vi "iRobot Navigation Target.vi"() -> ()   [LabVIEW 2015]
uses:
  iRobot/Sensor/OI Mode.ctl
  iRobot/Sensor/Charging Sources Available.ctl
  iRobot/Sensor/Cargo Bay Digital Inputs.ctl
  iRobot/Sensor/Charging State.ctl
  iRobot/Sensor/Buttons.ctl
  iRobot/Sensor/Low-Side Driver + Wheel Overcurrent.ctl
  iRobot/Sensor/Bumps + Wheel Drops.ctl
  <vilib>/Statechart/Infrastructure/RTStatechart/RunTime SCN.xnode
  iRobot/Sensor/Sensor Group 6.ctl
  Accelerometer.ctl
  iRobot Navigation State Machine.lvsc
  iRobot Navigation State Machine.lvsc/Inputs.ctl
  iRobot Navigation State Machine.lvsc/Outputs.ctl
  iRobot Navigation State Machine.lvsc/Trigger.ctl
  iRobot Navigation State Machine.lvsc/State.ctl
  iRobot Navigation State Machine.lvsc/StatechartState.ctl
  <vilib>/myRIO/Instrument Drivers/Utilities/Utilities.lvlib
  iRobot Navigation State Machine.lvsc/CompanionDiagram.vi
  iRobot Navigation State Machine.lvsc/CompanionDiagram.vi/52/SC Main.vi
  <vilib>/myRIO/Express VI/Onboard IO/I2C/I2C Express VI.xnode
  <vilib>/myRIO/Instrument Drivers/Onboard IO/I2C/vis/Configure.vi
  <vilib>/myRIO/Instrument Drivers/Onboard IO/I2C/I2C.lvlib
  <vilib>/myRIO/Instrument Drivers/Onboard IO/I2C/typedefs/I2C Transfer Rate.ctl
  <vilib>/myRIO/Instrument Drivers/Onboard IO/I2C/typedefs/I2C User Configuration.ctl
  <vilib>/myRIO/Instrument Drivers/Onboard IO/I2C/typedefs/I2C Configuration.ctl
  <vilib>/myRIO/Common/Instrument Driver Framework/myRIO v1.0/I2C/typedefs/I2C Channels Enum.ctl
  <vilib>/myRIO/Common/Instrument Driver Framework/Utilities/typedefs/Generic FPGA Reference.ctl
  <vilib>/myRIO/Common/Instrument Driver Framework/Utilities/typedefs/myRIO v1.0 Reference.ctl
  <vilib>/myRIO/Common/Instrument Driver Framework/Utilities/typedefs/Hardware Version Enum.ctl
  <vilib>/myRIO/Common/Instrument Driver Framework/Utilities/typedefs/myRIO Generic Hardware Reference.ctl
  <vilib>/myRIO/Instrument Drivers/Onboard IO/I2C/typedefs/I2C Reference.ctl
  <vilib>/myRIO/Instrument Drivers/Onboard IO/I2C/vis/myRIO I2C Open.xnode
  <vilib>/myRIO/Common/Instrument Driver Framework/Utilities/vis/Is FPGA Ref Available.vi
  <vilib>/myRIO/Common/Instrument Driver Framework/myRIO v1.0/I2C/vis/myRIO v1.1 Open I2C.vi
  <vilib>/userdefined/High Color/nirio_resource_hc.ctl
  iRobot Sensors.ctl
panel:
  out "StateData.Speed":i16
  in  "Tab Control":T1(tab)
  out "Right Wheel":i16
  out "Left Wheel":i16
  out "PID output":dbl
  in  "Kd Constant":dbl
  in  "Ki Constant":dbl=30.0
  in  "Kp Constant":dbl=350.0
  out "Current barcode time":dbl
  in  "Barcode Response\nTime Delay":dbl=0.5
  in  "Barcode Time Threshold \n(to measure lenght of each line":dbl=0.45
  in  "Barcode Tape \nSensor Threshold":u16=600
  out "iRobot Sensors (graphical)":T2 {"Right Wheel (mm/s)" scale=-500.0..500.0; "Left Wheel (mm/s)" scale=-500.0..500.0}
  in  "Edge Tape\nSensor Threshold":u16=600
  out "Barcode Array":i32[](array[numeric])
  out "Active States":T4
  out "error out":errorcluster
  in  "Wheel Speed (mm/s)":i16(slide)=100 scale=0.0..500.0
  in  "accel smoothing (0-1)":dbl=0.1
  in  "stop":bool
  out "Target Running":bool
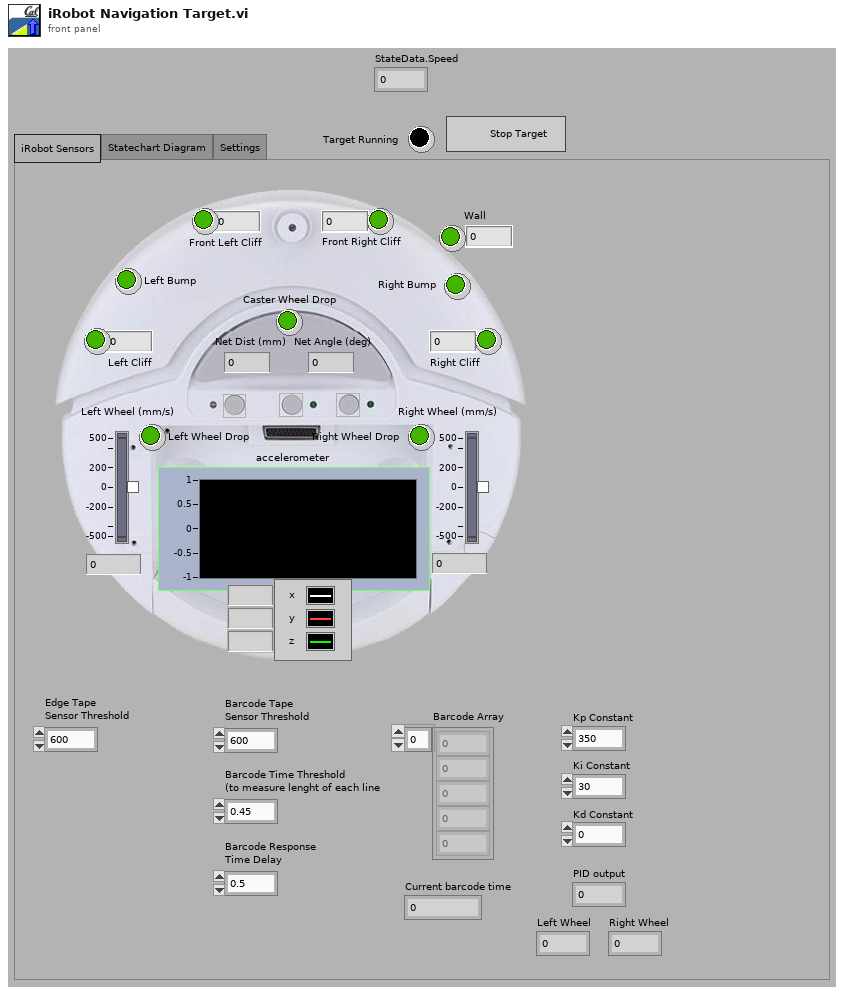
[diagram p1: front panel]
types:
  T1 = enum32{"iRobot Sensors", "Statechart Diagram", "Settings"}
  T2 = typedef "iRobot Sensors.ctl" = cluster{"Caster Wheel Drop":bool, "Left Wheel Drop":bool, "Right Wheel Drop":bool, "Left Bump":bool, "Right Bump":bool, "Left Cliff":bool, "Front Left Cliff":bool, "Front Right Cliff":bool, "Right Cliff":bool, "Wall":bool, "Net Dist (mm)":i32, "Net Angle (deg)":i32, "Wall":u16, "Left Cliff":u16, "Front Left Cliff":u16, "Front Right Cliff":u16, "Right Cliff":u16, "Left Wheel (mm/s)":i16, "Right Wheel (mm/s)":i16, "accelerometer":T3}
  T3 = typedef "Accelerometer.ctl" = cluster{"x axis (g)":dbl, "y axis (g)":dbl, "z axis (g)":dbl}
  T4 = typedef "iRobot Navigation State Machine.lvsc/StatechartState.ctl" = T5[]
  T5 = typedef "iRobot Navigation State Machine.lvsc/State.ctl" = enum16{"NI.SC.Initial", "NI.SC.History", "NI.SC.ShallowHistory", "NI.SC.Terminal", "Pause", "Run", "Pause\\Detect Play Button\\Pause;\nWait for\nbutton\nrelease", "Pause\\Detect Play Button\\Unpause;\nwait for\nbutton release", "Pause\\Detect Play Button\\Unpause;\nwait for\nbutton press", "Run\\Detect Obstacles\\Recover from head on\nedge collision", "Run\\Detect Obstacles\\Check barcode or edge", "Run\\Detect Obstacles\\Right Bumper", "Run\\Detect Obstacles\\Clear the barcode 2", "Run\\Detect Obstacles\\Clear the barcode", "Run\\Detect Obstacles\\Left Bumper", "Run\\Detect Obstacles\\Slow Down", "Run\\Detect Obstacles\\Speed Up", "Run\\Detect Obstacles\\Turn Right", "Run\\Detect Obstacles\\Turn Left", "Run\\Detect Obstacles\\Light", "Run\\Detect Obstacles\\Dark", "Run\\Detect Obstacles\\Straighten Left", "Run\\Detect Obstacles\\Straighten Right", "Run\\Detect Obstacles\\Barcode Drive", "Run\\Detect Obstacles\\Hit Right Boundary /\n Turn Left", "Run\\Detect Obstacles\\Hit Left Boundary / \nTurn Right", "Run\\Detect Obstacles\\Drive"}
  T6 = typedef "iRobot UART Port Type.ctl" = refnum<visa-resource-name>
  T7 = typedef "I2C.lvlib/I2C Reference.ctl" = cluster{"myRIO Reference":T8, "I2C Channels Enum":T12, "I2C Configuration":T13}
  T8 = typedef "myRIO Generic Hardware Reference.ctl" = cluster{"myRIO Model":T9, "myRIO Hardware Reference":T10}
  T9 = typedef "Hardware Version Enum.ctl" = enum16{"Unknown", "myRIO-1900", "myRIO-1950", "roboRIO"}
  T10 = typedef "myRIO v1.0 Reference.ctl" = cluster{"Generic FPGA Reference":T11, "Allow multiple opens":bool}
  T11 = typedef "Generic FPGA Reference.ctl" = refnum<k20>
  T12 = typedef "I2C Channels Enum.ctl" = enum16{"Not Connected", "A/I2C", "B/I2C", "I2C/I2C"}
  T13 = typedef "I2C.lvlib/I2C Configuration.ctl" = cluster{"I2C Transfer Rate":T14}
  T14 = typedef "I2C.lvlib/I2C Transfer Rate.ctl" = enum16{"Standard mode (100 kbps)", "Fast mode (400 kbps)"}
  T15 = typedef "I2C.lvlib/I2C User Configuration.ctl" = cluster{"I2C Transfer Rate":T14}
  T16 = typedef "nirio_resource_hc.ctl" = tag
  T17 = typedef "iRobot Navigation State Machine.lvsc/Inputs.ctl" = cluster{"net distance (mm)":i32, "net angle (deg)":i32, "Max Wheel Speed (mm/s)":i16, "accelerometer":T3, "iRobot Sensors":T18, "Is Simulator?":bool, "Edge Tape Threshold":u16, "Barcode Tape Threshold":u16, "Barcode Time Threshold":dbl, "Barcode Action Time":dbl, "Kp Constant":dbl, "Ki Constant":dbl, "Kd Constant":dbl}
  T18 = typedef "Sensor Group 6.ctl" = cluster{"Bumps + Wheel Drops":T19, "Wall":bool, "Cliff Left":bool, "Cliff Front Left":bool, "Cliff Front Right":bool, "Cliff Right":bool, "Virtual Wall":bool, "Low-Side Driver + Wheel Overcurrent":T20, "Infrared":u8, "Buttons":T21, "Distance (mm)":i32, "Angle (deg)":i32, "Charging State":T22, "Voltage (mV)":u16, "Current (mA)":i16, "Battery Temperature (deg C)":i8, "Battery Charge (mAh)":u16, "Battery Capacity (mAh)":u16, "Wall Signal (0-4095)":u16, "Cliff Left Signal (0-4095)":u16, "Cliff Front Left Signal (0-4095)":u16, "Cliff Front Right Signal (0-4095)":u16, "Cliff Right Signal (0-4095)":u16, "Cargo Bay Digital Inputs":T23, "Cargo Bay Analog Signal (0-1023)":u16, "Charging Sources Available":T24, "OI Mode":T25, "Song Number":u8, "Song Playing":bool, "Number of Stream Packets":u8, "Requested Velocity (mm/s)":i16, "Requested Radius (mm)":i16, "Requested Right Wheel Velocity (mm/s)":i16, "Requested Left Wheel Velocity (mm/s)":i16}
  T19 = typedef "Bumps + Wheel Drops.ctl" = cluster{"Wheeldrop Caster":bool, "Wheeldrop Left":bool, "Wheeldrop Right":bool, "Bump Left":bool, "Bump Right":bool}
  T20 = typedef "Low-Side Driver + Wheel Overcurrent.ctl" = cluster{"Low-Side Driver 0":bool, "Low-Side Driver 1":bool, "Low-Side Driver 2":bool, "Left Wheel":bool, "Right Wheel":bool}
  T21 = typedef "Buttons.ctl" = cluster{"Advance":bool, "Play":bool}
  T22 = typedef "Charging State.ctl" = enum16{"Not Charging", "Reconditioning Charging", "Full Charging", "Trickle Charging", "Waiting", "Charging Fault Condition"}
  T23 = typedef "Cargo Bay Digital Inputs.ctl" = cluster{"Digital Input 0":bool, "Digital Input 1":bool, "Digital Input 2":bool, "Digital Input 3":bool, "Device Detect":bool}
  T24 = typedef "Charging Sources Available.ctl" = cluster{"Internal Charger":bool, "Home Base":bool}
  T25 = typedef "OI Mode.ctl" = enum16{"Off", "Passive", "Safe", "Full"}
  T26 = typedef "iRobot Navigation State Machine.lvsc/Outputs.ctl" = cluster{"Left Wheel Speed (mm/s)":i16, "Right Wheel Speed (mm/s)":i16, "Current time":dbl, "Array":i32[], "PID output":dbl, "Left wheel":i16, "Right wheel":i16, "StateData.Speed":i16}
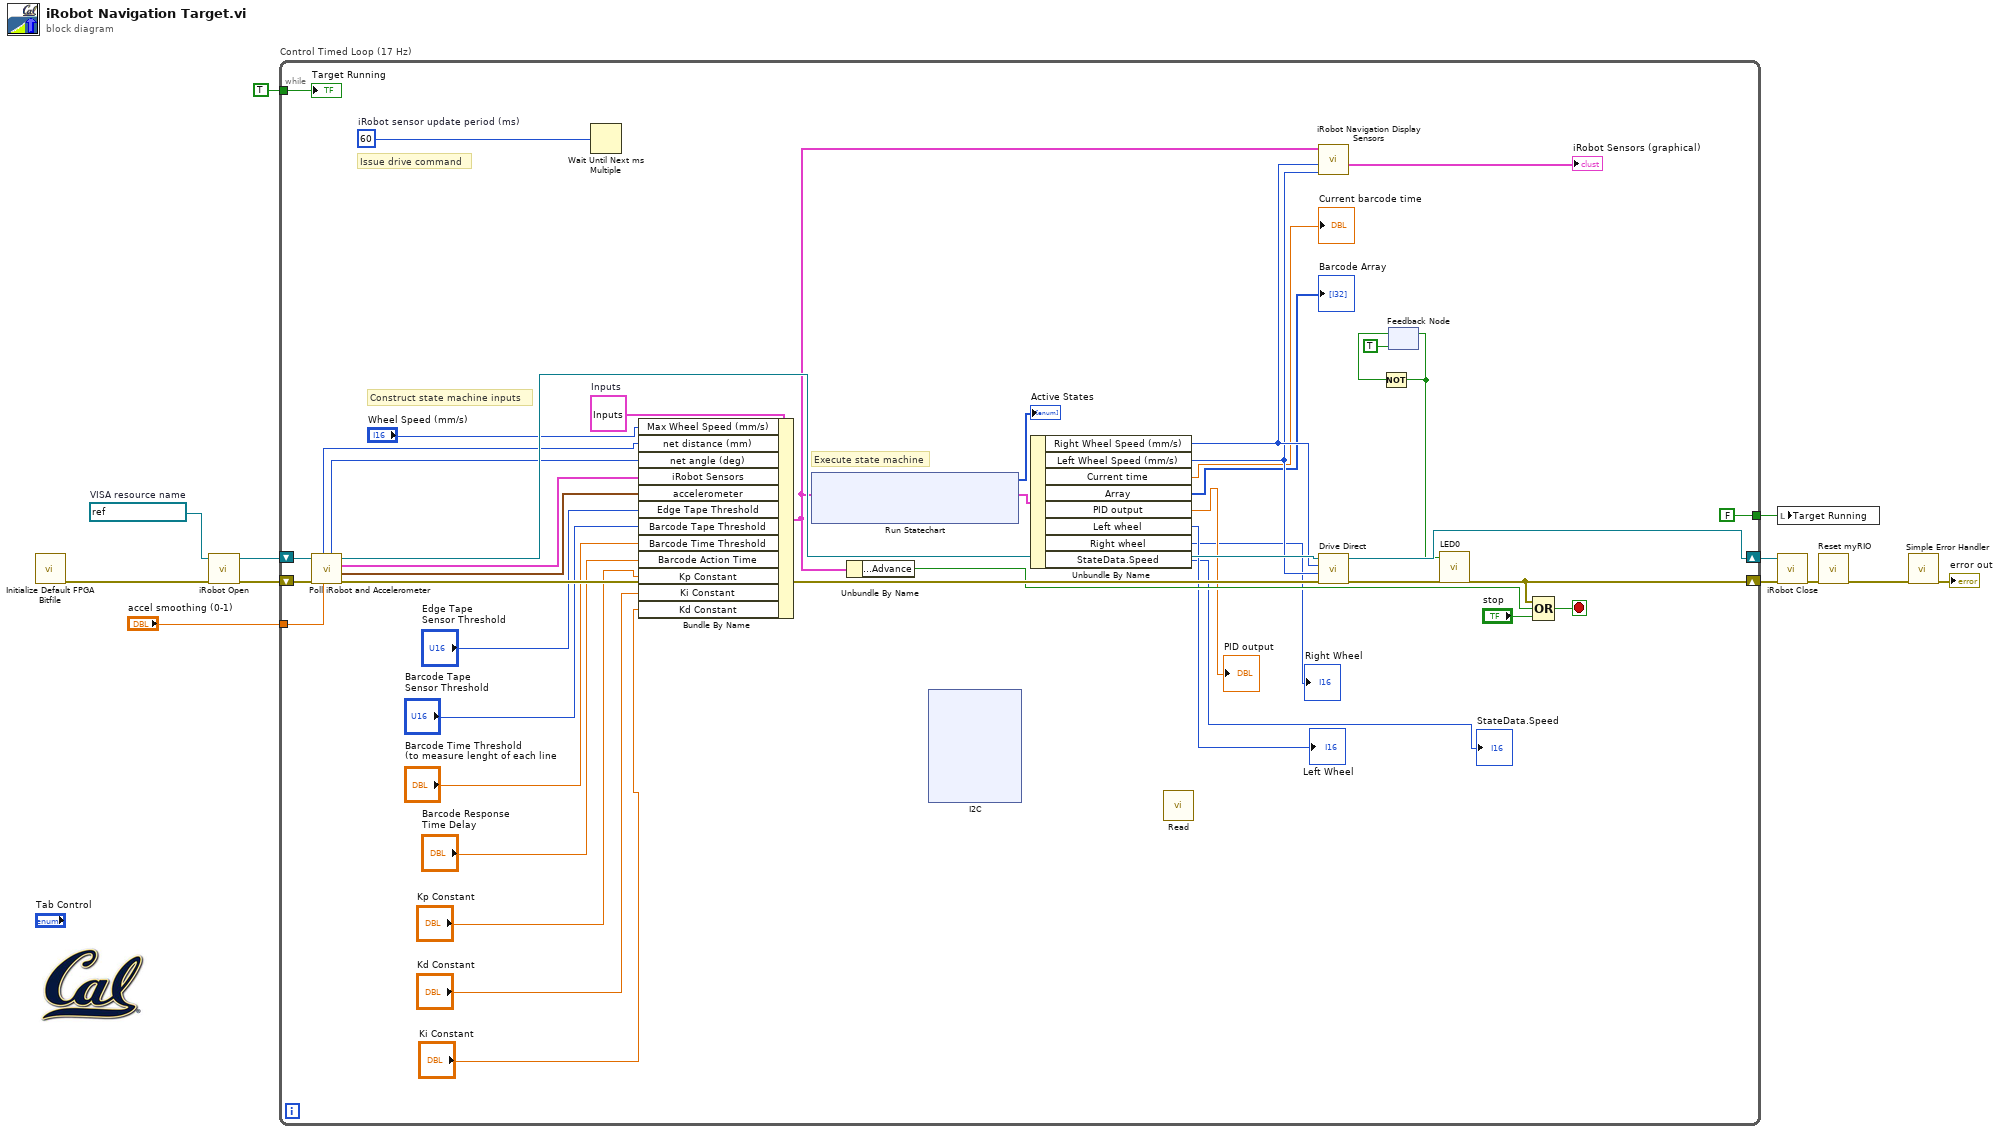
[diagram p0: block diagram]
diagram:
  w6 = refnum<visa-resource-name> "ASRL1::INSTR"  # VISA resource name
  n1 = call <vilib>:"Initialize Default FPGA Bitfile.vi"() -> ("error out"=w4:errorcluster)  [unwired: 11 in]
  n2 = call "iRobot Open.vi"("error in (no error)"=w4, "UART port in"=w6) -> ("error out"=w11:errorcluster, "UART port out"=w10:T6)  [unwired: 8 in]
  n3 = while "Control Timed Loop (17 Hz)" {
    shift-right: [w54] -> w12
    shift-left: w10 -> [w49]
    shift-right: [w36] -> w7
    shift-left: w11 -> [w48]
    tunnel: TRUE ("stop") -> [w42]
    tunnel: [FALSE ("stop")] -> w8
    tunnel: "accel smoothing (0-1)" -> [w28]
    stop <- w53 stop-if-true
    w26 = u32 60  # iRobot sensor update period (ms)
    w51 = T17 {"net distance (mm)"=0, "net angle (deg)"=0, "Max Wheel Speed (mm/s)"=0, "accelerometer"={"x axis (g)"=0.0, "y axis (g)"=0.0, "z axis (g)"=0.0}, "iRobot Sensors"={"Bumps + Wheel Drops"={"Wheeldrop Caster"=FALSE, "Wheeldrop Left"=FALSE, "Wheeldrop Right"=FALSE, "Bump Left"=FALSE, "Bump Right"=FALSE}, "Wall"=FALSE, "Cliff Left"=FALSE, "Cliff Front Left"=FALSE, "Cliff Front Right"=FALSE, "Cliff Right"=FALSE, "Virtual Wall"=FALSE, "Low-Side Driver + Wheel Overcurrent"={"Low-Side Driver 0"=FALSE, "Low-Side Driver 1"=FALSE, "Low-Side Driver 2"=FALSE, "Left Wheel"=FALSE, "Right Wheel"=FALSE}, "Infrared"=255, "Buttons"={"Advance"=FALSE, "Play"=FALSE}, "Distance (mm)"=0, "Angle (deg)"=0, "Charging State"=enum."Not Charging", "Voltage (mV)"=0, "Current (mA)"=0, "Battery Temperature (deg C)"=0, "Battery Charge (mAh)"=0, "Battery Capacity (mAh)"=0, "Wall Signal (0-4095)"=0, "Cliff Left Signal (0-4095)"=0, "Cliff Front Left Signal (0-4095)"=0, "Cliff Front Right Signal (0-4095)"=0, "Cliff Right Signal (0-4095)"=0, "Cargo Bay Digital Inputs"={"Digital Input 0"=FALSE, "Digital Input 1"=FALSE, "Digital Input 2"=FALSE, "Digital Input 3"=FALSE, "Device Detect"=FALSE}, "Cargo Bay Analog Signal (0-1023)"=0, "Charging Sources Available"={"Internal Charger"=FALSE, "Home Base"=FALSE}, "OI Mode"=enum."Off", "Song Number"=0, "Song Playing"=FALSE, "Number of Stream Packets"=0, "Requested Velocity (mm/s)"=0, "Requested Radius (mm)"=0, "Requested Right Wheel Velocity (mm/s)"=0, "Requested Left Wheel Velocity (mm/s)"=0}, "Is Simulator?"=FALSE, "Edge Tape Threshold"=0, "Barcode Tape Threshold"=0, "Barcode Time Threshold"=0.0, "Barcode Action Time"=0.0, "Kp Constant"=0.0, "Ki Constant"=0.0, "Kd Constant"=0.0}  # Inputs
    # "Issue drive command"
    # "Execute state machine"
    # "Construct state machine inputs"
    n4 = call "Poll iRobot and Accelerometer.vi"("accel smoothing (0-1)"=w28, "error in"=w48, "UART port in"=w49) -> ("error out"=w47:errorcluster, "Acceleration (g)"=w27:T3, "iRobot SensorGroup6"=w35:T18, "UART port out"=w46:T6, "net angle (deg)"=w44:i32, "net distance (mm)"=w45:i32)  [unwired: 3 in]
    n5 = Wait Until Next ms Multiple(millisecond multiple=w26) -> ()  [unwired: 1 out]
    n6 = Bundle By Name(cluster=w51, "Max Wheel Speed (mm/s)"="Wheel Speed (mm/s)", "net distance (mm)"=w45, "net angle (deg)"=w44, "iRobot Sensors"=w35, "accelerometer"=w27, "Edge Tape Threshold"="Edge Tape\nSensor Threshold", "Barcode Tape Threshold"="Barcode Tape \nSensor Threshold", "Barcode Time Threshold"="Barcode Time Threshold \n(to measure lenght of each line", "Barcode Action Time"="Barcode Response\nTime Delay", "Kp Constant"="Kp Constant", "Ki Constant"="Kd Constant", "Kd Constant"="Ki Constant") -> (w30:T17)
    n7 = xnode "Run Statechart"("Inputs"=w30) -> ("Outputs"=w52:T26, "Active States"=→"Active States":T4)  [unwired: 2 in, 1 out]
    n8 = Unbundle By Name(w30) -> ("iRobot Sensors.Buttons.Advance"=w29:bool)
    n9 = xnode "I2C"() -> ()  [unwired: 3 in, 2 out]
    n10 = Unbundle By Name(w52) -> ("Right Wheel Speed (mm/s)"=w33:i16, "Left Wheel Speed (mm/s)"=w32:i16, "Current time"=→"Current barcode time":dbl, "Array"=→"Barcode Array":i32[], "PID output"=→"PID output":dbl, "Left wheel"=→"Left Wheel":i16, "Right wheel"=→"Right Wheel":i16, "StateData.Speed"=→"StateData.Speed":i16)
    n11 = call <vilib>:"Read.vi"() -> ()  [unwired: 8 in, 3 out]
    n12 = call "iRobot Navigation Display Sensors.vi"("Left Wheel (mm/s)"=w32, "Right Wheel (mm/s)"=w33, "Statechart Inputs"=w30) -> ("iRobot Sensors (graphical)"=→"iRobot Sensors (graphical)":T2)  [unwired: 6 in]
    n13 = call "Drive Direct.vi"("error in"=w47, "Left Wheel Velocity (mm/s)"=w32, "Right Wheel Velocity (mm/s)"=w33, "UART port in"=w46) -> ("error out"=w37:errorcluster, "UART port out"=w54:T6)  [unwired: 6 in]
    n14 = feedback #1(TRUE) -> (w38:bool)
    n15 = Not(x=w38) -> (.not. x?=w39:bool)
    n16 = feedback-in #1(w39) -> ()
    n17 = call "LED0"("LED0"=w39, "error in (no error)"=w37) -> ("error out"=w36:errorcluster)  [unwired: 25 in]
    n18 = Compound Arithmetic op=OR(w36, w29, "stop") -> (w53:bool)
    "Target Running" <- w42
  }
  n19 = local write "Target Running"(w8) -> ()
  n20 = call "iRobot Close.vi"("error in"=w7, "UART port in"=w12) -> ("error out"=w1:errorcluster)  [unwired: 9 in]
  n21 = call <vilib>:"Reset myRIO.vi"("error in (no error)"=w1) -> ("error out"=w5:errorcluster)  [unwired: 10 in]
  n22 = call <vilib>:"Simple Error Handler.vi"("error in (no error)"=w5) -> ("error out"=→"error out":errorcluster)  [unwired: 4 in, 4 out]
